vi "Test_Assert32BitOrLessInt_UnbrokenFor32BitOrLess.vi"(8 "error in (no error)":errorcluster, 11 "TestCase in":refnum<class "Test Assertions.lvclass">) -> (0 "error out":errorcluster, 3 "TestCase out":refnum<class "Test Assertions.lvclass">)   [LabVIEW 2020, in "Test Assertions.lvclass"]
uses:
  <vilib>/gpm_packages/composed-database-configuration/externals/assertions/Test/Test Assertions/Test Assertions.lvclass
  <vilib>/addons/_JKI Toolkits/VI Tester/TestCase.llb/TestCase.lvclass
  C:/Program Files/National Instruments/LabVIEW 2020/vi.lib/addons/_JKI Toolkits/VI Tester/TestCase.llb/TestCase.lvclass
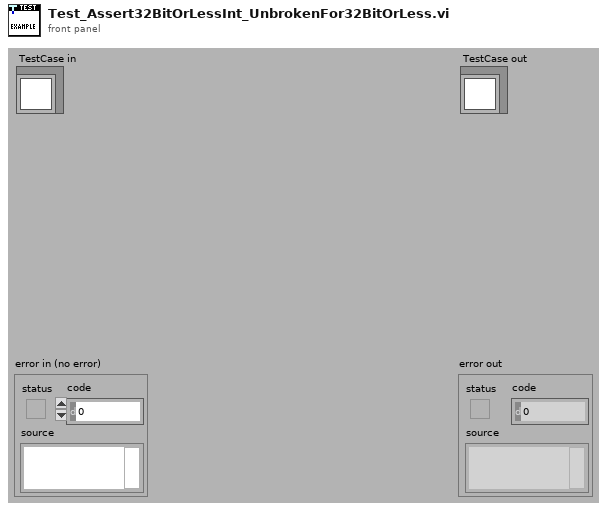
[diagram p1: front panel]
types:
  T1 = enum32{"Bad", "Idle", "Run top level", "Running"}
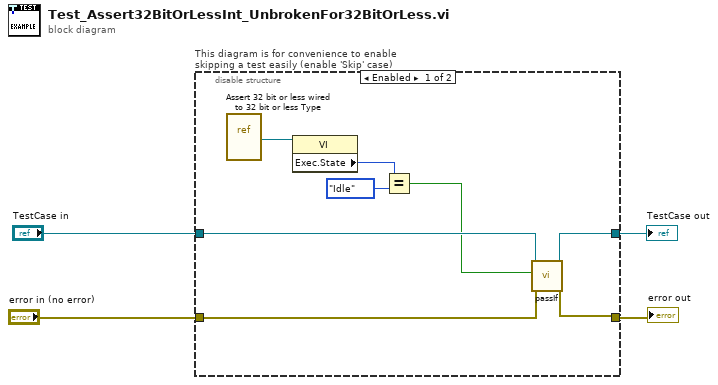
[diagram p0: block diagram]
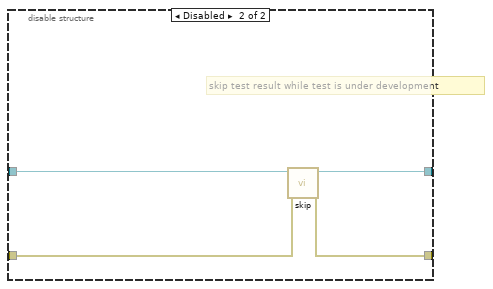
[diagram p2: hidden frame]
diagram:
  n1 = disable-structure "This diagram is for convenience to enable skipping a test easily (enable 'Skip' case)" shown="Enabled" {
    disable-tunnel: "TestCase in" -> [w12 w16]
    disable-tunnel: [w11 w14] -> w1
    disable-tunnel: [w10 w15] -> w3
    disable-tunnel: "error in (no error)" -> [w9 w13]
    frame Enabled {
      n2 = vi-ref <vilib>:"Assert 32 bit or less wired to 32 bit or less Type.vi"() -> (w8:refnum<vi>)
      n3 = property class="VI"(reference=w8) -> ("Exec.State"=w7:T1)  [unwired: 1 in, 2 out]
      n4 = Equal?(x=w7, y=T1."Idle") -> (x = y?=w5:bool)
      n5 = call-dynamic "passIf.vi"("error in (no error)"=w9, "pass"=w5, "TestCase in"=w12) -> ("error out"=w10:errorcluster, "TestCase out"=w11:refnum<class "Test Assertions.lvclass">)  [unwired: 7 in]
    }
    frame Disabled {
      # "skip test result while test is under development"
      n6 = call <vilib>:"skip.vi"("error in (no error)"=w13, "TestCase in"=w16) -> ("error out"=w15:errorcluster, "TestCase out"=w14:refnum<class "Test Assertions.lvclass">)  [unwired: 8 in]
    }
  }
  "error out" <- w3
  "TestCase out" <- w1
